vi "CmdSet_Cmd_OMAN.vi"(10 "cmd in":string) -> (2 "cmd out":string)   [LabVIEW 8.6]
panel:
  in  "bin":cluster{"x":i16, "y":i16}
  in  "roi":cluster{"xc":i16, "yc":i16, "xl":i16, "yl":i16}
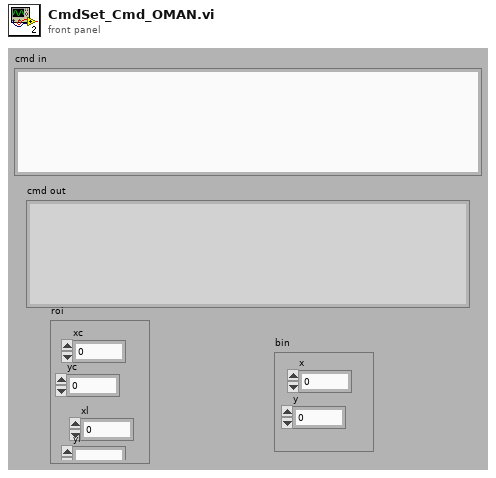
[diagram p1: front panel]
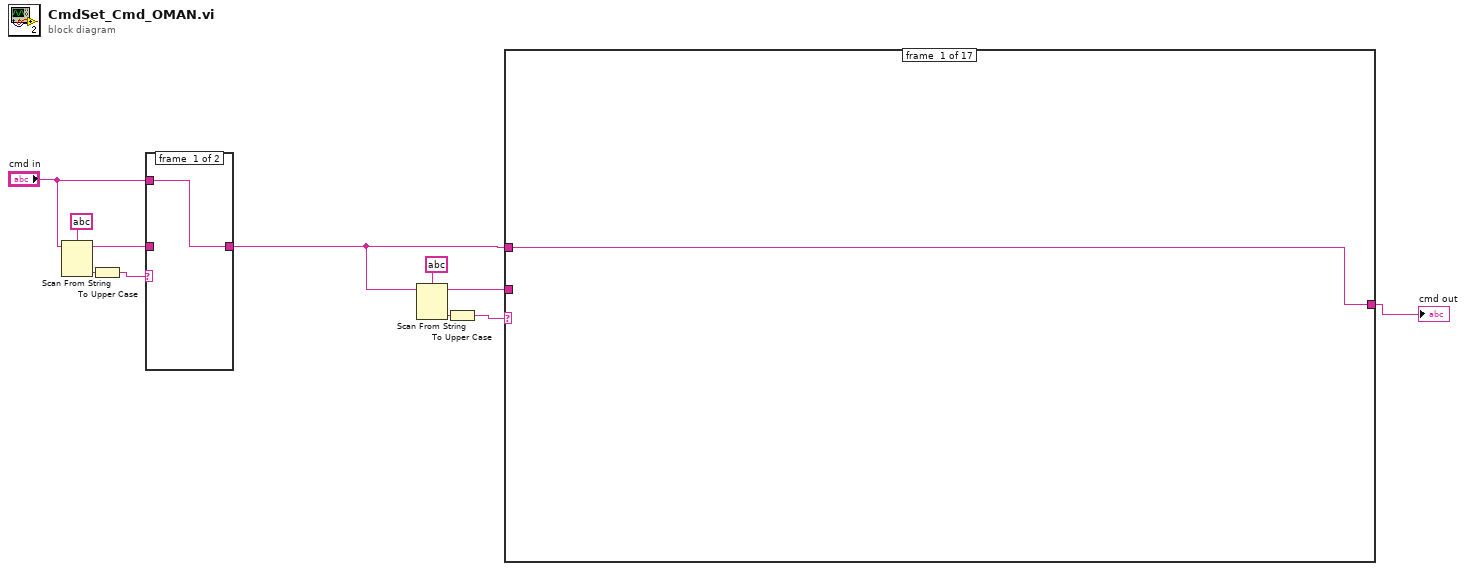
[diagram p0: block diagram]
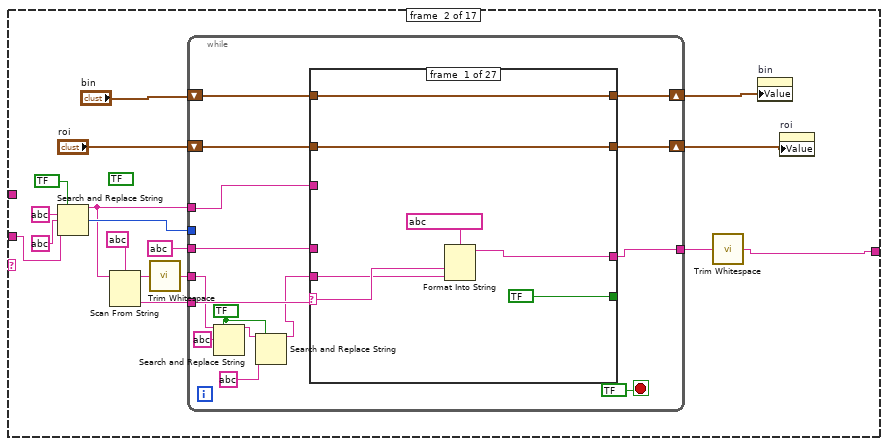
[diagram p2: hidden frame]
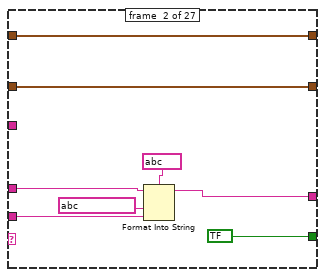
[diagram p3: hidden frame]
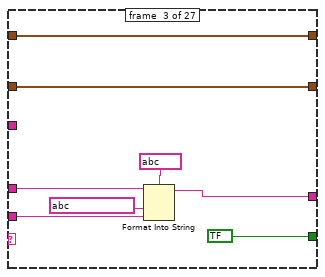
[diagram p4: hidden frame]
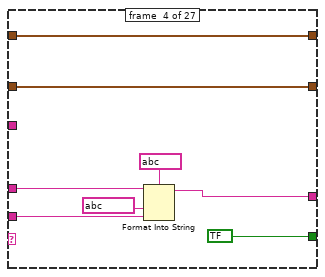
[diagram p5: hidden frame]
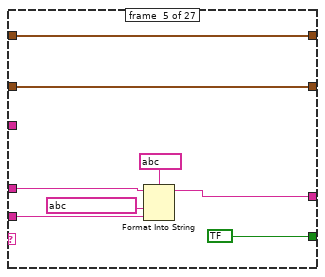
[diagram p6: hidden frame]
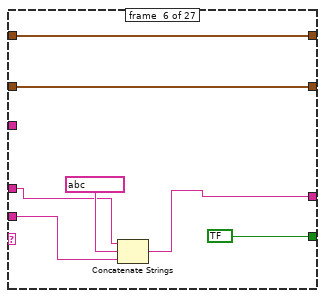
[diagram p7: hidden frame]
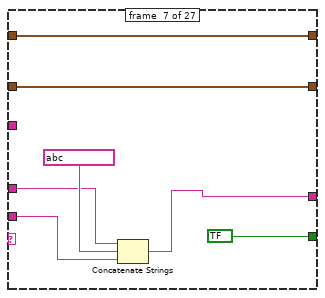
[diagram p8: hidden frame]
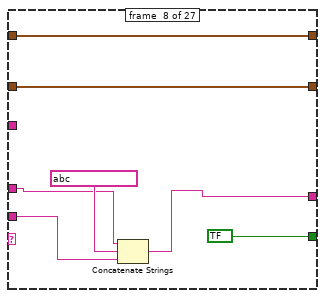
[diagram p9: hidden frame]
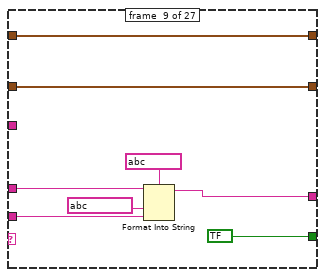
[diagram p10: hidden frame]
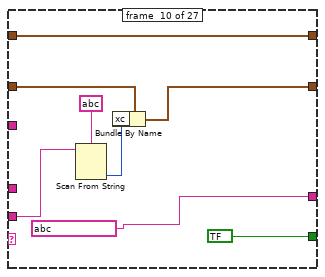
[diagram p11: hidden frame]
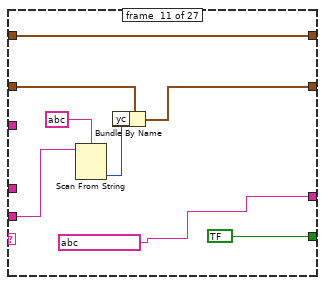
[diagram p12: hidden frame]
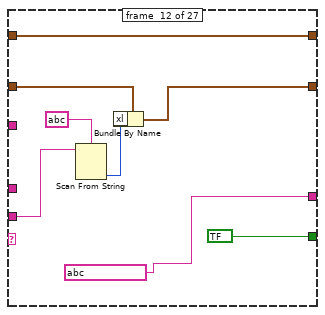
[diagram p13: hidden frame]
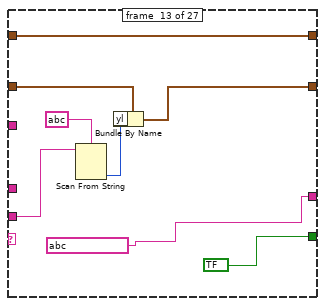
[diagram p14: hidden frame]
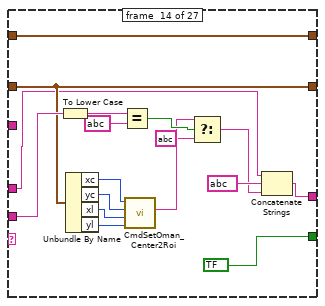
[diagram p15: hidden frame]
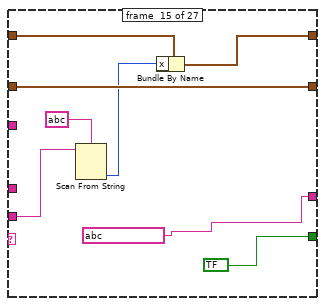
[diagram p16: hidden frame]
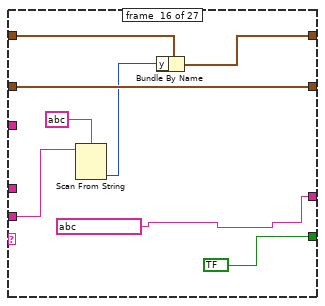
[diagram p17: hidden frame]
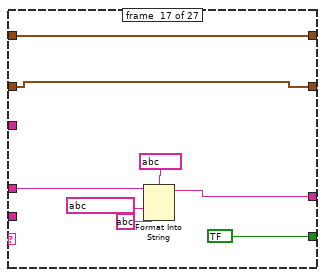
[diagram p18: hidden frame]
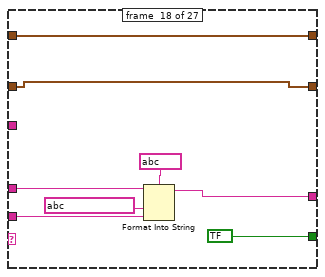
[diagram p19: hidden frame]
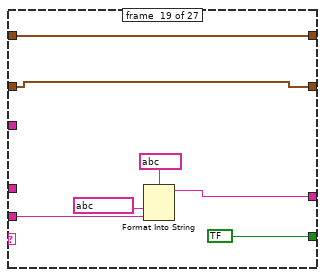
[diagram p20: hidden frame]
diagram:
  n1 = Scan From String(format string=string ?, input string="cmd in") -> (remaining string=w8:string, output 1=w10:string)  [unwired: 2 in, 3 out]
  n2 = To Upper Case(1:w10) -> (0:w9:string)
  n3 = case shown="\"DHE\"" w9 {
    tunnel: w8 -> [_ w14]
    tunnel: [w12 w13] -> w1
    tunnel: "cmd in" -> [w12 _]
    frame #0 {
    }
    frame #1 {
      n4 = call <vilib>:"Trim Whitespace.vi"("string"=w14) -> ("trimmed string"=w13:string)  [unwired: 1 in]
    }
  }
  n5 = Scan From String(format string=string ?, input string=w1) -> (remaining string=w3:string, output 1=w6:string)  [unwired: 2 in, 3 out]
  n6 = To Upper Case(1:w6) -> (0:w4:string)
  n7 = case shown="\"EXPPARAMS\"" w4 {
    tunnel: [w15 w21 w249 w257 string ? ("trimmed string") w264 w272 string ? ("trimmed string") string ? ("trimmed string") string ? ("trimmed string") w279 string ? ("trimmed string") string ? ("trimmed string") string ? ("trimmed string") string ? ("trimmed string") string ? ("trimmed string") w290] -> w2
    tunnel: w3 -> [_ w29 w243 _ _ w263 w269 _ _ _ w278 _ _ _ _ _ w294]
    tunnel: w1 -> [w15 _ _ _ _ _ _ _ _ _ _ _ _ _ _ _ _]
    frame #0 {
    }
    frame #1 {
      (unwired) bool ? ("replace all? (F)")
      n8 = Search and Replace String(replace all?=bool ? ("replace all? (F)"), input string=w29, search string=string ?, replace string=string ? ("replace string (\"\")")) -> (result string=w27:string, number of replacements=w28:i32)  [unwired: 1 in, 5 out]
      n9 = Scan From String(format string=string ?, input string=w27) -> (remaining string=w24:string, output 1=w25:string)  [unwired: 2 in, 3 out]
      n10 = call <vilib>:"Trim Whitespace.vi"("string"=w24) -> ("trimmed string"=w23:string)  [unwired: 1 in]
      n11 = while {
        shift-right: [w46] -> w16
        shift-left: "roi" -> [w47]
        shift-right: [w44] -> w17
        shift-left: "bin" -> [w45]
        tunnel: w28 -> [_]
        tunnel: w27 -> [w42]
        tunnel: w25 -> [w41]
        tunnel: w23 -> [w38]
        tunnel: [w40] -> w22
        tunnel: string ? -> [w39]
        stop <- bool ? stop-if-true
        w33 = bool ? ("replace all? (F)")
        n12 = Search and Replace String(replace all?=w33, input string=w38, search string=string ?) -> (result string=w36:string)  [unwired: 2 in, 6 out]
        n13 = Search and Replace String(replace all?=w33, input string=w36, search string=string ?) -> (result string=w34:string)  [unwired: 2 in, 6 out]
        n14 = case shown="\"STATE\"" w41 {
          selector: w41 -> [w51 _ _ _ _ _ _ _ _ _ _ _ _ _ _ _ _ _ _ _ _ _ _ _ _ w235 _]
          tunnel: w34 -> [w50 w59 w67 w75 w83 w89 w96 w102 w112 w120 w128 w136 w145 w157 w171 w179 _ w193 w200 _ _ _ _ _ w226 w234 _]
          tunnel: [bool ? bool ? bool ? bool ? bool ? bool ? bool ? bool ? bool ? bool ? bool ? bool ? bool ? bool ? bool ? bool ? bool ? bool ? bool ? bool ? bool ? bool ? bool ? bool ? bool ? bool ? bool ?] -> _
          tunnel: [w53 w61 w69 w77 w85 w88 w95 w103 w114 string ? ("string") string ? ("string") string ? ("string") string ? ("string") w158 string ? ("string") string ? ("string") w187 w195 w202 string ? string ? ("string") string ? ("string") string ? ("string") string ? ("string") w224 w232 string ?] -> w40
          tunnel: w47 -> [w49 w57 w65 w73 w81 w92 w99 w106 w110 w122 w130 w138 w146 w150 w169 w177 w184 w191 w198 w206 w210 w214 w218 w222 w229 w237 w240]
          tunnel: [w49 w57 w65 w73 w81 w92 w99 w106 w110 w121 w129 w137 w143 w150 w169 w177 w184 w191 w198 w206 w210 w214 w218 w222 w229 w237 w240] -> w46
          tunnel: w45 -> [w48 w56 w64 w72 w80 w91 w98 w105 w109 w117 w125 w133 w141 w160 w168 w176 w183 w190 w197 w205 w209 w213 w217 w221 w228 w236 w239]
          tunnel: [w48 w56 w64 w72 w80 w91 w98 w105 w109 w117 w125 w133 w141 w160 w167 w175 w183 w190 w197 w205 w209 w213 w217 w221 w228 w236 w239] -> w44
          tunnel: w42 -> [_ _ _ _ _ _ _ _ _ _ _ _ _ _ _ _ _ _ _ _ _ _ _ _ _ _ _]
          tunnel: w39 -> [_ w55 w63 w71 w79 w87 w94 w101 w108 _ _ _ _ w148 _ _ w181 w189 _ _ _ _ _ _ _ _ _]
          frame #0 {
            n15 = Format Into String(format string=string ?, w51, w50) -> (resulting string=w53:string)  [unwired: 2 in, 1 out]
          }
          frame #1 {
            n16 = Format Into String(format string=string ?, initial string=w55, string ? ("input 1"), w59) -> (resulting string=w61:string)  [unwired: 1 in, 1 out]
          }
          frame #2 {
            n17 = Format Into String(format string=string ?, initial string=w63, string ? ("input 1"), w67) -> (resulting string=w69:string)  [unwired: 1 in, 1 out]
          }
          frame #3 {
            n18 = Format Into String(format string=string ?, initial string=w71, string ? ("input 1"), w75) -> (resulting string=w77:string)  [unwired: 1 in, 1 out]
          }
          frame #4 {
            n19 = Format Into String(format string=string ?, initial string=w79, string ? ("input 1"), w83) -> (resulting string=w85:string)  [unwired: 1 in, 1 out]
          }
          frame #5 {
            n20 = Concatenate Strings(w87, string ? ("input 1"), w89) -> (w88:string)
          }
          frame #6 {
            n21 = Concatenate Strings(w94, string ? ("input 1"), w96) -> (w95:string)
          }
          frame #7 {
            n22 = Concatenate Strings(w101, string ? ("input 1"), w102) -> (w103:string)
          }
          frame #8 {
            n23 = Format Into String(format string=string ?, initial string=w108, string ? ("input 1"), w112) -> (resulting string=w114:string)  [unwired: 1 in, 1 out]
          }
          frame #9 {
            n24 = Scan From String(format string=string ?, input string=w120) -> (output 1=w118:i32)  [unwired: 2 in, 4 out]
            n25 = Bundle By Name(cluster=w122, "xc"=w118) -> (w121:cluster{"xc":i16, "yc":i16, "xl":i16, "yl":i16})
          }
          frame #10 {
            n26 = Scan From String(format string=string ?, input string=w128) -> (output 1=w126:i32)  [unwired: 2 in, 4 out]
            n27 = Bundle By Name(cluster=w130, "yc"=w126) -> (w129:cluster{"xc":i16, "yc":i16, "xl":i16, "yl":i16})
          }
          frame #11 {
            n28 = Scan From String(format string=string ?, input string=w136) -> (output 1=w134:i32)  [unwired: 2 in, 4 out]
            n29 = Bundle By Name(cluster=w138, "xl"=w134) -> (w137:cluster{"xc":i16, "yc":i16, "xl":i16, "yl":i16})
          }
          frame #12 {
            n30 = Scan From String(format string=string ?, input string=w145) -> (output 1=w142:i32)  [unwired: 2 in, 4 out]
            n31 = Bundle By Name(cluster=w146, "yl"=w142) -> (w143:cluster{"xc":i16, "yc":i16, "xl":i16, "yl":i16})
          }
          frame #13 {
            n32 = To Lower Case(string=w157) -> (all lower case string=w155:string)
            n33 = Unbundle By Name(w150) -> ("xc"=w163:i16, "yc"=w162:i16, "xl"=w161:i16, "yl"=w149:i16)
            n34 = Equal?(x=w155, y=string ?) -> (x = y?=w154:bool)
            n35 = call "CmdSetOman_Center2Roi.vi"("yl"=w149, "xl"=w161, "yc"=w162, "xc"=w163) -> ("roi"=w153:string)  [unwired: 7 out]
            n36 = Select(t=w153, s=w154, f=string ?) -> (s? t:f=w151:string)
            n37 = Concatenate Strings(w148, string ? ("string"), w151) -> (w158:string)
          }
          frame #14 {
            n38 = Scan From String(format string=string ?, input string=w171) -> (output 1=w166:i32)  [unwired: 2 in, 4 out]
            n39 = Bundle By Name(cluster=w168, "x"=w166) -> (w167:cluster{"x":i16, "y":i16})
          }
          frame #15 {
            n40 = Scan From String(format string=string ?, input string=w179) -> (output 1=w174:i32)  [unwired: 2 in, 4 out]
            n41 = Bundle By Name(cluster=w176, "y"=w174) -> (w175:cluster{"x":i16, "y":i16})
          }
          frame #16 {
            n42 = Format Into String(format string=string ?, initial string=w181, string ? ("input 1"), string ? ("input 2")) -> (resulting string=w187:string)  [unwired: 1 in, 1 out]
          }
          frame #17 {
            n43 = Format Into String(format string=string ?, initial string=w189, string ? ("input 1"), w193) -> (resulting string=w195:string)  [unwired: 1 in, 1 out]
          }
          frame #18 {
            n44 = Format Into String(format string=string ?, string ? ("input 1"), w200) -> (resulting string=w202:string)  [unwired: 2 in, 1 out]
          }
          frame #19 {
          }
          frame #20 {
          }
          frame #21 {
          }
          frame #22 {
          }
          frame #23 {
          }
          frame #24 {
            n45 = case shown="\"15\", Default" w226 {
              tunnel: [string ?] -> w225
              frame "15", Default {
              }
            }
            n46 = Concatenate Strings(string ? ("string"), w225) -> (w224:string)
          }
          frame #25 {
            n47 = call <vilib>:"Space Constant.vi"() -> ("String"=w233:string)
            n48 = Concatenate Strings(w235, w233, w234) -> (w232:string)
          }
          frame #26 {
          }
        }
      }
      n49 = call <vilib>:"Trim Whitespace.vi"("string"=w22) -> ("trimmed string"=w21:string)  [unwired: 1 in]
      n50 = property on="bin" class="Clust (strict)"("Value"=w17) -> ()  [unwired: 2 in, 2 out]
      n51 = property on="roi" class="Clust (strict)"("Value"=w16) -> ()  [unwired: 2 in, 2 out]
    }
    frame #2 {
      n52 = Scan From String(format string=string ?, input string=w243) -> (output 1=w247:string)  [unwired: 2 in, 4 out]
      n53 = property on="roi" class="Clust (strict)"() -> ("Value"=w251:cluster{"xc":i16, "yc":i16, "xl":i16, "yl":i16})  [unwired: 2 in, 2 out]
      n54 = Unbundle By Name(w251) -> ("xc"=w254:i16, "yc"=w253:i16, "xl"=w252:i16, "yl"=w244:i16)
      n55 = call "CmdSetOman_Center2Roi.vi"("yl"=w244, "xl"=w252, "yc"=w253, "xc"=w254) -> ("roi"=w246:string)  [unwired: 7 out]
      n56 = case shown="Default" w247 {
        tunnel: w246 -> [_ w256]
        tunnel: [string ? ("roi") w256] -> w245
        frame #0 {
        }
        frame #1 {
        }
      }
      n57 = Concatenate Strings(string ? ("string"), w245) -> (w249:string)
    }
    frame #3 {
      n58 = property on="bin" class="Clust (strict)"() -> ("Value"=w261:cluster{"x":i16, "y":i16})  [unwired: 2 in, 2 out]
      n59 = Unbundle By Name(w261) -> ("x"=w260:i16, "y"=w259:i16)
      n60 = Format Into String(format string=string ?, w260, w259) -> (resulting string=w257:string)  [unwired: 2 in, 1 out]
    }
    frame #4 {
    }
    frame #5 {
      n61 = Scan From String(format string=string ?, input string=w263) -> (output 1=w265:string)  [unwired: 2 in, 4 out]
      n62 = case shown="Default" w265 {
        tunnel: [string ? ("trimmed string") string ? ("trimmed string")] -> w264
        frame #0 {
        }
        frame #1 {
        }
      }
    }
    frame #6 {
      n63 = Scan From String(format string=string ?, input string=w269) -> (output 1=w270:string)  [unwired: 2 in, 4 out]
      n64 = case shown="\"EXP_PROG\", \"EXP_PROG2\"" w270 {
        tunnel: [string ? ("trimmed string") string ? ("trimmed string")] -> w272
        frame #0 {
        }
        frame #1 {
        }
      }
    }
    frame #7 {
    }
    frame #8 {
    }
    frame #9 {
    }
    frame #10 {
      n65 = Scan From String(format string=string ?, input string=w278) -> (output 1=w281:string)  [unwired: 2 in, 4 out]
      n66 = To Lower Case(string=w281) -> (all lower case string=w280:string)
      n67 = case shown="\"open\"" w280 {
        tunnel: [string ? ("trimmed string") string ? ("trimmed string")] -> w279
        frame #0 {
        }
        frame #1 {
        }
      }
    }
    frame #11 {
    }
    frame #12 {
    }
    frame #13 {
    }
    frame #14 {
    }
    frame #15 {
    }
    frame #16 {
      n68 = Scan From String(format string=string ?, input string=w294) -> (output 1=w291:string)  [unwired: 2 in, 4 out]
      n69 = Format Into String(format string=string ?, w291) -> (resulting string=w290:string)  [unwired: 2 in, 1 out]
    }
  }
  "cmd out" <- w2
